vi "Custom Packet Single.vi"() -> ()   [LabVIEW 2021]
uses:
  <userlib>/SciSDK/SciSDK_Labview.lvlib
panel:
  out "Counter 3":u32
  out "Counter 2":u32
  out "Counter 1":u32
  out "Counter 0":u32
  out "Timestamp":u32
  out "Header":string
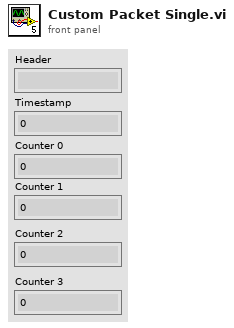
[diagram p1: front panel]
types:
  T1 = cluster{"Name":string, "Board Model":string, "Handle":u64}
  T2 = cluster{"Board Name":string, "Board Model":string, "SciSDK Handle":u64}
  T3 = cluster{"packet_size":u32, "buffer_size":u32, "magic":u32, "valid_data":dbl, "data":u32[]}
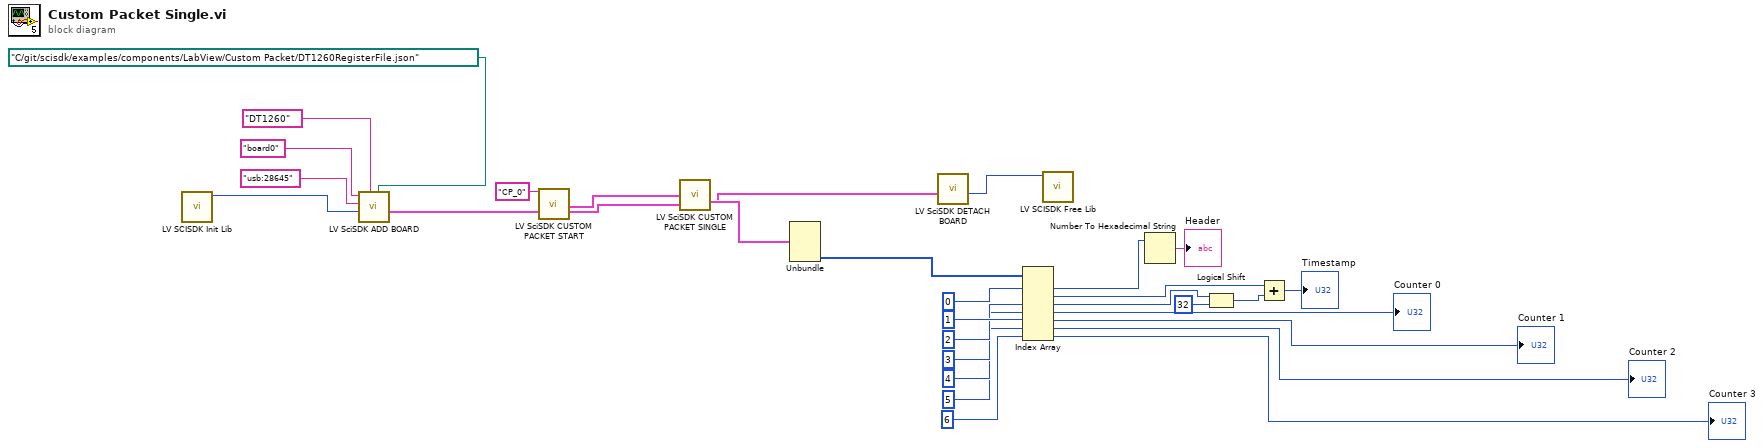
[diagram p0: block diagram]
diagram:
  n1 = call <userlib>:"LV SCISDK Init Lib.vi"() -> ("function return"=w31:u64)  [unwired: 11 in]
  n2 = call <userlib>:"LV SciSDK ADD BOARD.vi"("JsonFile"=path "C:/git/scisdk/examples/components/LabView/Custom Packet/DT1260RegisterFile.json", "Board Model"="DT1260", "SciSDK Handle"=w31, "DevicePath"="usb:28645", "Name"="board0") -> ("Board Handle Out"=w26:T1)  [unwired: 4 in, 2 out]
  n3 = call <userlib>:"LV SciSDK CUSTOM PACKET START.vi"("Custom Packet Name"="CP_0", "Handle In"=w26) -> ("CP Handle Out"=w5:cluster{"CP Path":string, "CP Name":string}, "Board Handle Out"=w6:T2)  [unwired: 15 in, 1 out]
  n4 = call <userlib>:"LV SciSDK CUSTOM PACKET SINGLE.vi"("CP Handle In"=w5, "Handle In"=w6) -> ("CP Buffer Out"=w4:T3, "Handle Out"=w2:T2)  [unwired: 9 in, 3 out]
  n5 = Unbundle(w4) -> ("data"=w3:u32[])  [unwired: 4 out]
  n6 = call <userlib>:"LV SciSDK DETACH BOARD.vi"("Board Handle In"=w2) -> ("SciSDK Handle"=w1:u64)  [unwired: 9 in, 1 out]
  n7 = Index Array(array=w3, index #1=0 ("index"), index #2=1 ("index"), index #3=2 ("index"), index #4=3 ("index"), index #5=4 ("index"), index #6=5 ("index"), index #7=6 ("index")) -> (element #1=w17:u32, element #2=w12:u32, element #3=w14:u32, element #4=→"Counter 0":u32, element #5=→"Counter 1":u32, element #6=→"Counter 2":u32, element #7=→"Counter 3":u32)
  n8 = call <userlib>:"LV SCISDK Free Lib.vi"("handle"=w1) -> ()  [unwired: 9 in, 2 out]
  n9 = Number To Hexadecimal String(2:w17) -> (0:→"Header":string)  [unwired: 1 in]
  n10 = Logical Shift(y=w14, x=u32 32) -> (x << y=w13:u32)
  n11 = Add(x=w12, y=w13) -> (x+y=→"Timestamp":u32)
